vi "UHR-Fleezers Control (host) - 12.5.vi"() -> ()   [LabVIEW 2012] (continued)
                                n602 = Wait (ms)(milliseconds to wait=u32 700) -> ()  [unwired: 1 out]
                                }
                                frame #2 {
                                n603 = local read "Action (%)"() -> (w916:dbl)
                                n604 = Absolute Value(x=w916) -> (abs(x)=w915:dbl)
                                n605 = Greater?(x=w915, y=70.0) -> (0:w913:bool)
                                n606 = property on="Remove Action Offset" class="Bool (strict)"("Val(Sgnl)"=w913) -> ()  [unwired: 2 in, 2 out]
                                }
                                frame #3 {
                                n607 = for {
                                N: 4 -> [_]
                                n608 = flat-sequence {
                                frame #0 {
                                n609 = Wait (ms)(milliseconds to wait=u32 500) -> ()  [unwired: 1 out]
                                }
                                frame #1 {
                                n610 = local read "Action (%)"() -> (w922:dbl)
                                n611 = Absolute Value(x=w922) -> (abs(x)=w921:dbl)
                                n612 = Greater?(x=w921, y=70.0) -> (0:w919:bool)
                                n613 = property on="Remove Action Offset" class="Bool (strict)"("Val(Sgnl)"=w919) -> ()  [unwired: 2 in, 2 out]
                                }
                                }
                                }
                                }
                                frame #4 {
                                n614 = local read "Shift confocal"() -> (w927:bool)
                                n615 = local read "Mean"() -> (w929:dbl)
                                n616 = Greater?(x=w929, y=11.0) -> (0:w926:bool)
                                n617 = Not(x=w926) -> (.not. x?=w925:bool)
                                n618 = And(x=w926, y=w927) -> (x .and. y?=w924:bool)
                                n619 = And(x=w925, y=w927) -> (x .and. y?=w923:bool)
                                n620 = case shown="True" w924 {
                                frame False {
                                }
                                frame True {
                                n621 = local read "Confocal Y 2 (V)"() -> (w933:dbl)
                                n622 = local read "Confocal X 2 (V)"() -> (w932:dbl)
                                n623 = property on="AO2" class="Slide (strict)"("Val(Sgnl)"=w932) -> ()  [unwired: 2 in, 2 out]
                                n624 = property on="AO1" class="Slide (strict)"("Val(Sgnl)"=w933) -> ()  [unwired: 2 in, 2 out]
                                }
                                }
                                n625 = case shown="True" w923 {
                                frame False {
                                }
                                frame True {
                                n626 = local read "Confocal X 1 (V)"() -> (w930:dbl)
                                n627 = local read "Confocal Y 1 (V)"() -> (w931:dbl)
                                n628 = property on="AO1" class="Slide (strict)"("Val(Sgnl)"=w931) -> ()  [unwired: 2 in, 2 out]
                                n629 = property on="AO2" class="Slide (strict)"("Val(Sgnl)"=w930) -> ()  [unwired: 2 in, 2 out]
                                }
                                }
                                }
                                frame #5 {
                                n630 = Wait (ms)(milliseconds to wait=u32 1500) -> ()  [unwired: 1 out]
                                }
                                frame #6 {
                                n631 = property on="Rem fb disp offset" class="Bool (strict)"("Val(Sgnl)"=TRUE ("Value (Signaling)")) -> ()  [unwired: 2 in, 2 out]
                                }
                                }
                                }
                                frame True {
                                n632 = flat-sequence {
                                tunnel: w936 -> [w937]
                                frame #0 {
                                n633 = property on="Trap Delta (MHz)" class="DigNum (strict)"("Val(Sgnl)"=w937) -> ()  [unwired: 2 in, 2 out]
                                }
                                frame #1 {
                                n634 = Wait (ms)(milliseconds to wait=u32 500) -> ()  [unwired: 1 out]
                                }
                                frame #2 {
                                n635 = local read "Shift confocal"() -> (w943:bool)
                                n636 = local read "Mean"() -> (w945:dbl)
                                n637 = Greater?(x=w945, y=11.0) -> (0:w942:bool)
                                n638 = Not(x=w942) -> (.not. x?=w941:bool)
                                n639 = And(x=w942, y=w943) -> (x .and. y?=w940:bool)
                                n640 = And(x=w941, y=w943) -> (x .and. y?=w939:bool)
                                n641 = case shown="True" w940 {
                                frame False {
                                }
                                frame True {
                                n642 = local read "Confocal Y 2 (V)"() -> (w949:dbl)
                                n643 = local read "Confocal X 2 (V)"() -> (w948:dbl)
                                n644 = property on="AO2" class="Slide (strict)"("Val(Sgnl)"=w948) -> ()  [unwired: 2 in, 2 out]
                                n645 = property on="AO1" class="Slide (strict)"("Val(Sgnl)"=w949) -> ()  [unwired: 2 in, 2 out]
                                }
                                }
                                n646 = case shown="True" w939 {
                                frame False {
                                }
                                frame True {
                                n647 = local read "Confocal Y 1 (V)"() -> (w947:dbl)
                                n648 = local read "Confocal X 1 (V)"() -> (w946:dbl)
                                n649 = property on="AO2" class="Slide (strict)"("Val(Sgnl)"=w946) -> ()  [unwired: 2 in, 2 out]
                                n650 = property on="AO1" class="Slide (strict)"("Val(Sgnl)"=w947) -> ()  [unwired: 2 in, 2 out]
                                }
                                }
                                }
                                }
                                }
                                }
                                }
                                }
                                }
                                }
                                n651 = local read "Messages"() -> (w895:string)
                                n652 = Subtract(x=w887, y=w886) -> (x-y=w893:dbl)
                                "Duration (s)" <- w893
                                n653 = Number To Decimal String(number=w893, width (-)=i16 0) -> (decimal integer string=w891:string)
                                n654 = Concatenate Strings(w891, " s fluorescence event." ("string")) -> (w889:string)
                                n655 = call "Update messages.vi"("Message to add"=w889, "Old message string"=w895) -> ("New message string"=w894:string)
                                n656 = local write "Reset Force"(FALSE ("Reset Force")) -> ()
                                n657 = local write "Waiting"(TRUE ("Waiting")) -> ()
                                n658 = local write "Messages"(w894) -> ()
                                n659 = local write "Fl. High"(FALSE ("Fl. High")) -> ()
                                n660 = call <vilib>:"Beep.vi"() -> ()  [unwired: 3 in, 9 out]
                                }
                                }
                                n661 = node-c288() -> ()  [unwired: 2 out]
                              }
                              n662 = node-c288(w863) -> ()  [unwired: 1 out]
                            }
                          }
                        }
                      }
                      n663 = local read "Trap Delta (MHz)"() -> (w778:dbl)
                      n664 = local read "Trap Pos FB SP"() -> (w773:fxp<+/-,16,1>)
                    }
                  }
                }
                frame #1 {
                  n665 = local read "Stop All"() -> (w959:bool)
                  n666 = local read "Fl. Triggered..."() -> (w957:bool)
                  n667 = Not(x=w957) -> (.not. x?=w958:bool)
                  n668 = Or(x=w958, y=w959) -> (x .or. y?=w956:bool)
                }
              }
              n669 = case shown="True" w550 {
                frame False {
                }
                frame True {
                  n670 = local read "Confocal Y 1 (V)"() -> (w560:dbl)
                  n671 = local read "Confocal X 1 (V)"() -> (w559:dbl)
                  n672 = property on="AO2" class="Slide (strict)"("Val(Sgnl)"=w559) -> ()  [unwired: 2 in, 2 out]
                  n673 = property on="AO1" class="Slide (strict)"("Val(Sgnl)"=w560) -> ()  [unwired: 2 in, 2 out]
                }
              }
              n674 = case shown="True" w550 {
                frame False {
                }
                frame True {
                  w558 = FALSE ("Fl. High")
                  n675 = local write "Waiting"(w558) -> ()
                  n676 = local write "Fl. High"(w558) -> ()
                }
              }
              n677 = node-c288() -> ()  [unwired: 2 out]
            }
            n678 = node-c288(w548) -> ()  [unwired: 1 out]
          }
        }
      }
      event "Stop All": Value Change {
        n679 = event-data() -> ()  [unwired: 7 out]
        n680 = local read "Stop All"() -> (w964:bool)
      }
    }
    n681 = node-c288() -> ()  [unwired: 2 out]
  }
  n682 = timed-loop "Run Scripts, including: stage motion" {
    tunnel: w119 -> [w972]
    tunnel: w118 -> [w973]
    tunnel: [w973] -> w117
    tunnel: [w972] -> w116
    timing: w114 -> [_]
    timing-out: [_] -> w113
    tunnel: w100 -> [w971]
    tunnel: w101 -> [w970]
    tunnel: w72 -> [w967]
    tunnel: w71 -> [w966]
    tunnel: w70 -> [w968]
    tunnel: w69 -> [w969]
    tunnel: w2 -> [w965]
    stop <- w974 stop-if-true
    n683 = node-c288() -> ()  [unwired: 1 in, 1 out]
    n684 = event shown="[20] \"Stop All\": Value Change" {
      selector: _ -> [_ _ _ _ _ _ _ _ _ _ _ _ _ _ _ _ _ _ _ _ _]
      dyn-events: _ -> [_ _ _ _ _ _ _ _ _ _ _ _ _ _ _ _ _ _ _ _ _]
      timeout: _ -> [_ _ _ _ _ _ _ _ _ _ _ _ _ _ _ _ _ _ _ _ _]
      tunnel: ["Set Position" "Move to Position" _ _ _ _ "Read Harvard" _ _ _ _ _ _ "Got ADig bead" "Force FB Data\nScript" _ "Got DNA bead" "Take Stepping Data" _ "Take Detection Laser\nImage" _] -> _
      tunnel: [_ _ _ _ _ _ _ _ _ _ _ _ _ _ _ _ _ _ _ _ w1626] -> w974
      tunnel: w972 -> [w992 w1000 w1013 w1043 _ _ _ w1117 w1157 w1238 w1267 w1399 w1425 _ w1461 _ _ _ _ _ _]
      tunnel: w973 -> [w993 w1001 w1014 w1044 _ _ _ w1118 w1158 w1239 w1268 w1400 w1426 _ w1462 _ _ _ _ _ _]
      tunnel: w971 -> [_ _ _ _ _ _ w1102 _ _ _ _ _ _ _ _ _ _ _ _ _ _]
      tunnel: w970 -> [_ _ _ _ _ _ w1101 _ _ _ _ _ _ _ _ _ _ _ _ _ _]
      tunnel: w969 -> [_ _ _ _ _ _ _ _ _ _ _ _ _ _ _ _ _ _ _ _ _]
      tunnel: w968 -> [_ _ _ _ _ _ _ _ _ _ _ _ _ _ _ _ _ _ _ _ _]
      tunnel: w967 -> [_ _ _ _ _ _ _ _ _ _ _ _ _ _ _ _ _ _ _ _ _]
      tunnel: w966 -> [_ _ _ _ _ _ _ _ _ _ _ _ _ _ _ _ _ _ _ _ _]
      tunnel: w965 -> [_ _ _ _ w1071 w1092 _ _ _ _ _ _ _ _ _ _ _ _ _ _ w1625]
      event "Set Position", "Set Position 2", "Set Position 3", "Set Position 4", "Set Position 5", "Set Position 1": Value Change {
        n685 = event-data() -> ()  [unwired: 1 in, 5 out]
        n686 = Build Array("Set Position 1", "Set Position 2", "Set Position 3", "Set Position 4", "Set Position 5") -> (w991:bool[])
        n687 = Boolean Array To Number(Boolean array=w991) -> (number=w990:u32)
        n688 = Logarithm Base 2(1:w990) -> (0:w982:dbl)
        n689 = call "Read Stage Position.vi"("error in"=w992, "VISA resource name in"=w993) -> ("Current Position"=w997:cluster{dbl, dbl, dbl}, "error out"=w996:errorcluster)  [unwired: 2 out]
        n690 = Decrement(x="Position") -> (x-1=w980:dbl)
        n691 = Greater Or Equal?(x=w982, y=0.0) -> (x >= y?=w983:bool)
        n692 = Cluster To Array(cluster=w997) -> (array=w994:dbl[])
        n693 = local write "Stage Control Serial Error"(w996) -> ()
        n694 = Select(t=w982, s=w983, f=w980) -> (s? t:f=w979:dbl)
        n695 = Increment(x=w979) -> (x+1=w978:dbl)
        n696 = Build Array (concatenate)(w978, w994) -> (w977:dbl[])
        n697 = Replace Array Subset(array="Saved Stage Positions", new element=w977, index (row)=w979) -> (w995:dbl[][])  [unwired: 1 in]
        n698 = local write "Saved Stage Positions"(w995) -> ()
      }
      event "Move to Position": Value Change {
        n699 = event-data() -> ()  [unwired: 1 in, 5 out]
        n700 = flat-sequence {
          tunnel: w1001 -> [w1005]
          tunnel: w1000 -> [w1004]
          frame #0 {
            n701 = local read "Saved Stage Positions"() -> (w1007:dbl[][])
            n702 = local read "Position"() -> (w1006:dbl)
            n703 = local write "Stage Moving"(TRUE ("Stage Moving")) -> ()
            n704 = call "move to saved stage position.vi"("error in"=w1004, "Stage VISA resource name in"=w1005, "Position"=w1006, "Saved Stage Positions"=w1007) -> ("error out"=w1003:errorcluster)  [unwired: 1 out]
            n705 = local write "Stage Control Serial Error"(w1003) -> ()
          }
          frame #1 {
            n706 = call <vilib>:"Beep.vi"() -> ()  [unwired: 3 in, 9 out]
            n707 = local write "Stage Moving"(FALSE ("Stage Moving")) -> ()
          }
        }
      }
      event "Move Cap. 1 (DNA Bottom)": Value Change {
        n708 = event-data() -> ()  [unwired: 1 in, 5 out]
        n709 = local write "Move Cap. 1 (DNA Bottom)"(FALSE ("Move Cap. 1 (DNA Right)")) -> ()
        n710 = flat-sequence {
          tunnel: w1013 -> [w1016]
          tunnel: w1014 -> [w1017]
          tunnel: [w1017] -> w1011
          tunnel: [w1016] -> w1010
          tunnel: w1011 -> [w1019]
          tunnel: w1010 -> [w1018]
          frame #0 {
            n711 = property on="Sample Channel\nFlow" class="Bool (strict)"("Val(Sgnl)"="Cap 1 Samp Flow ON") -> ()  [unwired: 2 in, 2 out]
          }
          frame #1 {
            n712 = local read "Saved Stage Positions"() -> (w1029:dbl[][])
            n713 = local write "Stage Moving"(TRUE ("Stage Moving")) -> ()
            n714 = Array Subset(array=w1029, index (row)=0 ("index"), length (row)=1 ("length"), index (col)=1 ("index"), length (col)=3 ("length")) -> (w1026:dbl[][])
            n715 = Reshape Array(w1026, 3 ("dimension size")) -> (w1024:dbl[])
            n716 = Array To Cluster(array=w1024) -> (cluster=w1023:cluster{"[0]":dbl, "[1]":dbl, "[2]":dbl})
            n717 = call "Set Stage Position.vi"("Position"=w1023, "error in"=w1018, "VISA resource name in"=w1019) -> ("error out"=w1022:errorcluster)  [unwired: 2 out]
            n718 = local write "Stage Control Serial Error"(w1022) -> ()
          }
          frame #2 {
            n719 = local write "Stage Moving"(FALSE ("Stage Moving")) -> ()
            n720 = case shown="True" "Cap 1 Flow ON" {
              frame False {
              }
              frame True {
                n721 = property on="Inject Pump 1" class="Bool (strict)"("Val(Sgnl)"=TRUE ("Value (Signaling)")) -> ()  [unwired: 2 in, 2 out]
              }
            }
            n722 = call <vilib>:"Beep.vi"() -> ()  [unwired: 3 in, 9 out]
          }
          frame #3 {
            n723 = property on="Sample Channel\nFlow" class="Bool (strict)"("Val(Sgnl)"=FALSE ("Value (Signaling)")) -> ()  [unwired: 2 in, 2 out]
            n724 = local read "Cap. 2 BD T1?\n(ADig T1, DNA T2)"() -> (w1036:bool)
            n725 = case shown="True" w1036 {
              tunnel: "Cap 1 T ON" -> [w1038 w1039]
              frame False {
                n726 = property on="Trap 1 (ON/OFF)" class="Bool (strict)"("Val(Sgnl)"=w1038) -> ()  [unwired: 2 in, 2 out]
              }
              frame True {
                n727 = property on="Trap 2 (ON/OFF)" class="Bool (strict)"("Val(Sgnl)"=w1039) -> ()  [unwired: 2 in, 2 out]
              }
            }
            n728 = property on="Got DNA bead" class="Bool"("Key Focus"=TRUE) -> ()  [unwired: 2 in, 2 out]
          }
        }
      }
      event "Move Cap. 2 (ADig Top)": Value Change {
        n729 = event-data() -> ()  [unwired: 1 in, 5 out]
        n730 = local write "Move Cap. 2 (ADig Top)"(FALSE ("Move Cap. 2 (ADig Left)")) -> ()
        n731 = flat-sequence {
          tunnel: w1043 -> [w1046]
          tunnel: w1044 -> [w1047]
          tunnel: [w1047] -> w1041
          tunnel: [w1046] -> w1040
          tunnel: w1041 -> [w1050]
          tunnel: w1040 -> [w1049]
          frame #0 {
            n732 = property on="Sample Channel\nFlow" class="Bool (strict)"("Val(Sgnl)"="Cap 2 Samp Flow ON") -> ()  [unwired: 2 in, 2 out]
          }
          frame #1 {
            w1048 = FALSE ("Value (Signaling)")
            n733 = local read "Saved Stage Positions"() -> (w1060:dbl[][])
            n734 = local write "Stage Moving"(TRUE ("Stage Moving")) -> ()
            n735 = Array Subset(array=w1060, index (row)=1 ("index"), length (row)=1 ("length"), index (col)=1 ("index"), length (col)=3 ("length")) -> (w1057:dbl[][])
            n736 = Reshape Array(w1057, 3 ("dimension size")) -> (w1055:dbl[])
            n737 = property on="Trap 1 (ON/OFF)" class="Bool (strict)"("Val(Sgnl)"=w1048) -> ()  [unwired: 2 in, 2 out]
            n738 = property on="Trap 1 (ON/OFF)" class="Bool (strict)"("Val(Sgnl)"=w1048) -> ()  [unwired: 2 in, 2 out]
            n739 = Array To Cluster(array=w1055) -> (cluster=w1054:cluster{"[0]":dbl, "[1]":dbl, "[2]":dbl})
            n740 = call "Set Stage Position.vi"("Position"=w1054, "error in"=w1049, "VISA resource name in"=w1050) -> ("error out"=w1053:errorcluster)  [unwired: 2 out]
            n741 = local write "Stage Control Serial Error"(w1053) -> ()
          }
          frame #2 {
            n742 = local write "Stage Moving"(FALSE ("Stage Moving")) -> ()
            n743 = call <vilib>:"Beep.vi"() -> ()  [unwired: 3 in, 9 out]
            n744 = case shown="True" "Cap 2 Flow ON" {
              frame False {
              }
              frame True {
                n745 = property on="Inject Pump 3" class="Bool (strict)"("Val(Sgnl)"=TRUE ("Value (Signaling)")) -> ()  [unwired: 2 in, 2 out]
              }
            }
          }
          frame #3 {
            n746 = property on="Sample Channel\nFlow" class="Bool (strict)"("Val(Sgnl)"=FALSE ("Value (Signaling)")) -> ()  [unwired: 2 in, 2 out]
            n747 = case shown="False" "Cap. 2 BD T1?\n(ADig T1, DNA T2)" {
              tunnel: "Cap 2 T ON" -> [w1069 w1070]
              frame False {
                n748 = property on="Trap 2 (ON/OFF)" class="Bool (strict)"("Val(Sgnl)"=w1069) -> ()  [unwired: 2 in, 2 out]
              }
              frame True {
                n749 = property on="Trap 1 (ON/OFF)" class="Bool (strict)"("Val(Sgnl)"=w1070) -> ()  [unwired: 2 in, 2 out]
              }
            }
            n750 = property on="Got ADig bead" class="Bool"("Key Focus"=TRUE) -> ()  [unwired: 2 in, 2 out]
          }
        }
      }
      event "Initialize Blue Laser": Value Change {
        n751 = event-data() -> ()  [unwired: 1 in, 5 out]
        n752 = flat-sequence {
          tunnel: w1071 -> [w1090]
          frame #0 {
            n753 = Concatenate Strings("slmp ", "Modulation\nPower (mW)") -> (w1089:string)
            n754 = call "serial write macro.vi"("String"=w1089, "Delay (ms)"="Delay (ms)", "VISA resource name"=w1090) -> ("read buffer"=w1078:string, "error out"=w1079:errorcluster, "VISA resource name out"=w1086:refnum<visa-resource-name>)
            n755 = local write "read blue buffer"(w1078) -> ()
            n756 = local write "Blue Error Out"(w1079) -> ()
            n757 = call "serial write macro.vi"("String"="sdmes 1", "Delay (ms)"="Delay (ms)", "VISA resource name"=w1086) -> ("read buffer"=w1076:string, "error out"=w1077:errorcluster, "VISA resource name out"=w1084:refnum<visa-resource-name>)
            n758 = local write "Blue Error Out"(w1077) -> ()
            n759 = local write "read blue buffer"(w1076) -> ()
            n760 = call "serial write macro.vi"("String"="sames 1", "Delay (ms)"="Delay (ms)", "VISA resource name"=w1084) -> ("read buffer"=w1073:string, "error out"=w1075:errorcluster, "VISA resource name out"=w1081:refnum<visa-resource-name>)
            n761 = local write "read blue buffer"(w1073) -> ()
            n762 = local write "Blue Error Out"(w1075) -> ()
            n763 = call "serial write macro.vi"("String"="l1", "Delay (ms)"="Delay (ms)", "VISA resource name"=w1081) -> ("read buffer"=w1072:string, "error out"=w1074:errorcluster)  [unwired: 1 out]
            n764 = local write "read blue buffer"(w1072) -> ()
            n765 = local write "Blue Error Out"(w1074) -> ()
          }
          frame #1 {
            n766 = local write "Initialize Blue Laser"(FALSE ("Initialize")) -> ()
          }
        }
      }
      event "Send string\nto Blue Laser": Value Change {
        n767 = event-data() -> ()  [unwired: 1 in, 5 out]
        n768 = flat-sequence {
          tunnel: w1092 -> [w1097]
          frame #0 {
            n769 = local read "Delay (ms)"() -> (w1094:i32)
            n770 = call "serial write macro.vi"("String"="command string", "Delay (ms)"=w1094, "VISA resource name"=w1097) -> ("read buffer"=w1095:string, "error out"=→"Blue Error Out":errorcluster)  [unwired: 1 out]
            "read blue buffer" <- w1095
            n771 = String Length(string=w1095) -> (length=→"length":i32)
            "command string sent" <- "command string"
          }
          frame #1 {
            n772 = local write "Send string\nto Blue Laser"(FALSE ("Send string")) -> ()
          }
        }
      }
      event "Read Harvard": Value Change {
        n773 = event-data() -> ()  [unwired: 1 in, 5 out]
        n774 = Concatenate Strings("write buffer", "\r") -> (w1104:string)
        n775 = VISA Write(VISA resource name=w1102, write buffer=w1104, error in (no error)=w1101) -> (VISA resource name out=w1113:refnum<visa-resource-name>, error out=w1112:errorcluster)  [unwired: 1 out]
        n776 = stacked-sequence {
          tunnel: [w1116] -> w1111
          tunnel: w1113 -> [w1116]
          tunnel: w1112 -> [w1115]
          tunnel: [w1115] -> w1106
          frame #0 {
            n777 = Wait (ms)(milliseconds to wait=50) -> ()  [unwired: 1 out]
          }
        }
        n778 = property class="Instr"(reference=w1111, error in=w1106) -> (reference out=w1110:refnum<visa-resource-name>, error out=w1108:errorcluster, "Serial Settings:Number of Bytes at Serial Port"=w1109:u32)
        "Serial Settings:Number of Bytes at Serial Port" <- w1109
        n779 = VISA Read(VISA resource name=w1110, byte count=w1109, error in (no error)=w1108) -> (read buffer=w1107:string)  [unwired: 3 out]
        "read buffer" <- w1107
        n780 = Fract/Exp String To Number(string=w1107) -> ()  [unwired: 5 out]
      }
      event "+z", "-z": Value Change {
        n781 = event-data() -> ()  [unwired: 1 in, 5 out]
        n782 = flat-sequence {
          tunnel: w1117 -> [w1139]
          tunnel: w1118 -> [w1119]
          frame #0 {
            n783 = call "Read Stage Position.vi"("error in"=w1139, "VISA resource name in"=w1119) -> ("Current Position"=w1124:cluster{dbl, dbl, dbl}, "error out"=w1137:errorcluster, "VISA resource name out"=w1138:refnum<visa-resource-name>)  [unwired: 1 out]
            n784 = local read "Saved Stage Positions"() -> (w1148:dbl[][])
            n785 = Divide(x="z nudge increment (um)", y=1000.0) -> (x/y=w1136:dbl)
            n786 = Boolean To (0,1)(Boolean="+z") -> (0, 1=w1128:i16)
            n787 = Boolean To (0,1)(Boolean="-z") -> (0, 1=w1129:i16)
            n788 = Array Subset(array=w1148, index (row)=1 ("index"), length (row)=1 ("length"), index (col)=1 ("index"), length (col)=3 ("length")) -> (w1145:dbl[][])
            n789 = Multiply(x=w1128, y=w1136) -> (x*y=w1132:dbl)
            n790 = Multiply(x=w1129, y=w1136) -> (x*y=w1130:dbl)
            n791 = Unbundle(w1124) -> (w1122:dbl, w1121:dbl, w1125:dbl)
            n792 = Negate(x=w1130) -> (-x=w1131:dbl)
            n793 = Reshape Array(w1145, 3 ("dimension size")) -> (w1143:dbl[])
            n794 = Add(x=w1132, y=w1131) -> (x+y=w1133:dbl)
            n795 = Array To Cluster(array=w1143) -> ()  [unwired: 1 out]
            n796 = Add(x=w1133, y=w1125) -> (x+y=w1123:dbl)
            n797 = Bundle(cluster=w1124, w1122, w1121, w1123) -> (w1120:cluster{dbl, dbl, dbl})
            n798 = call "Set Stage Position.vi"("Position"=w1120, "error in"=w1137, "VISA resource name in"=w1138) -> ("error out"=w1142:errorcluster)  [unwired: 2 out]
            n799 = local write "Stage Moving"(TRUE ("Stage Moving")) -> ()
            n800 = local write "Stage Control Serial Error"(w1142) -> ()
          }
          frame #1 {
            n801 = local write "Stage Moving"(FALSE ("Stage Moving")) -> ()
            n802 = call <vilib>:"Beep.vi"() -> ()  [unwired: 3 in, 9 out]
          }
        }
      }
      event "Cal/Data Acq. Spot": Value Change {
        n803 = event-data() -> ()  [unwired: 1 in, 5 out]
        n804 = flat-sequence {
          tunnel: w1157 -> [w1161]
          tunnel: w1158 -> [w1162]
          tunnel: [w1162] -> w1154
          tunnel: [w1161] -> w1153
          tunnel: w1154 -> [w1167]
          tunnel: w1153 -> [w1166]
          tunnel: ["Cal @ (MHz)"] -> w1151
          tunnel: [w1171] -> w1155
          tunnel: w1151 -> [w1171]
          tunnel: w1155 -> [w1180]
          tunnel: ["W/ Offset 1"] -> w1152
          tunnel: w1155 -> [w1201]
          tunnel: w1152 -> [w1199]
          frame #0 {
            n805 = property on="Sample Channel\nFlow" class="Bool (strict)"("Val(Sgnl)"="Daq spot flow on") -> ()  [unwired: 2 in, 2 out]
            n806 = Wait (ms)(milliseconds to wait=u32 250) -> ()  [unwired: 1 out]
          }
          frame #1 {
            n807 = local read "Saved Stage Positions"() -> (w1164:dbl[][])
            n808 = property on="Trap Delta (MHz)" class="DigNum (strict)"("Val(Sgnl)"="Cal @ (MHz)") -> ()  [unwired: 2 in, 2 out]
            n809 = local write "Stage Moving"(TRUE ("Stage Moving")) -> ()
            n810 = call "move to saved stage position.vi"("error in"=w1166, "Stage VISA resource name in"=w1167, "Position"="Cal Stage Position", "Saved Stage Positions"=w1164) -> ("error out"=w1165:errorcluster)  [unwired: 1 out]
            n811 = local write "Stage Control Serial Error"(w1165) -> ()
          }
          frame #2 {
            n812 = local write "Stage Moving"(FALSE ("Stage Moving")) -> ()
            n813 = property on="Sample Channel\nFlow" class="Bool (strict)"("Val(Sgnl)"="Flow ON during cal?") -> ()  [unwired: 2 in, 2 out]
            n814 = call <vilib>:"Beep.vi"() -> ()  [unwired: 3 in, 9 out]
          }
          frame #3 {
            n815 = Wait (ms)(milliseconds to wait=u32 1000) -> ()  [unwired: 1 out]
          }
          frame #4 {
            n816 = property on="Save Calibration" class="Bool (strict)"("Val(Sgnl)"=TRUE ("Value (Signaling)")) -> ()  [unwired: 2 in, 2 out]
          }
          frame #5 {
            n817 = Wait (ms)(milliseconds to wait=u32 2000) -> ()  [unwired: 1 out]
          }
          frame #6 {
            # "Check to see if \nsaving done"
            n818 = while {
              stop <- w1176 stop-if-true
              n819 = local read "Saving..."() -> (w1177:bool)
              n820 = Wait (ms)(milliseconds to wait=u32 100) -> ()  [unwired: 1 out]
              n821 = Not(x=w1177) -> (.not. x?=w1176:bool)
            }
          }
          frame #7 {
            n822 = case shown="True" "W/ Offset 1" {
              tunnel: w1180 -> [_ w1181]
              frame False {
              }
              frame True {
                n823 = stacked-sequence {
                  tunnel: w1181 -> [_ _ _ _ _ _ _ w1198]
                  frame #0 {
                    n824 = property on="Trap Delta (MHz)" class="DigNum (strict)"("Val(Sgnl)"="Offset 1 Start (MHz)") -> ()  [unwired: 2 in, 2 out]
                    n825 = Replace Array Subset(array=u32[] [0] ("Index Values"), new element="Offset 1 Set", index=0) -> (w1182:u32[])
                    n826 = property on="Saved AOD Raster Scan Parameter Sets" class="Arr (strict)"("Index Values"=w1182) -> ()  [unwired: 2 in, 2 out]
                  }
                  frame #1 {
                    n827 = Wait (ms)(milliseconds to wait=u32 200) -> ()  [unwired: 1 out]
                  }
                  frame #2 {
                    n828 = property on="Load parameters" class="Bool (strict)"("Val(Sgnl)"=TRUE ("Value (Signaling)")) -> ()  [unwired: 2 in, 2 out]
                  }
                  frame #3 {
                    n829 = Wait (ms)(milliseconds to wait=u32 200) -> ()  [unwired: 1 out]
                  }
                  frame #4 {
                    n830 = property on="Trap Raster Scan" class="Bool (strict)"("Val(Sgnl)"=TRUE ("Value (Signaling)")) -> ()  [unwired: 2 in, 2 out]
                  }
                  frame #5 {
                    n831 = Wait (ms)(milliseconds to wait=u32 2000) -> ()  [unwired: 1 out]
                  }
                  frame #6 {
                    n832 = while {
                      stop <- w1195 stop-if-true
                      n833 = local read "Raster Scanning..."() -> (w1197:bool)
                      n834 = local read "Saving..."() -> (w1193:bool)
                      n835 = Wait (ms)(milliseconds to wait=u32 100) -> ()  [unwired: 1 out]
                      n836 = Not(x=w1193) -> (.not. x?=w1192:bool)
                      n837 = Not(x=w1197) -> (.not. x?=w1194:bool)
                      n838 = And(x=w1194, y=w1192) -> (x .and. y?=w1195:bool)
                    }
                  }
                  frame #7 {
                    n839 = property on="Trap Delta (MHz)" class="DigNum (strict)"("Val(Sgnl)"=w1198) -> ()  [unwired: 2 in, 2 out]
                  }
                }
              }
            }
          }
          frame #8 {
            n840 = local read "Save ave N"() -> (w1200:dbl)
            n841 = case shown="False" "W/ Offset 2" {
              tunnel: w1201 -> [_ w1208]
              tunnel: w1200 -> [_ w1207]
              tunnel: w1199 -> [w1203 _]
              frame False {
                n842 = case shown="False" w1203 {
                  frame False {
                    n843 = Multiply(x="Cal read wait (s)", y=u32 1000 ("milliseconds to wait")) -> (x*y=w1205:u32)
                    n844 = Wait (ms)(milliseconds to wait=w1205) -> ()  [unwired: 1 out]
                  }
                  frame True {
                  }
                }
              }
              frame True {
                n845 = stacked-sequence {
                  tunnel: w1208 -> [_ _ _ _ _ _ _ _ _ w1229 _ _]
                  tunnel: w1207 -> [_ _ _ _ _ _ _ _ _ w1227 _ _]
                  frame #0 {
                    n846 = property on="Save ave N" class="DigNum (strict)"("Val(Sgnl)"=1.0 ("Value (Signaling)")) -> ()  [unwired: 2 in, 2 out]
                  }
                  frame #1 {
                    n847 = Wait (ms)(milliseconds to wait=u32 500) -> ()  [unwired: 1 out]
                  }
                  frame #2 {
                    n848 = property on="Trap Delta (MHz)" class="DigNum (strict)"("Val(Sgnl)"="Offset 2 Start (MHz)") -> ()  [unwired: 2 in, 2 out]
                    n849 = Replace Array Subset(array=u32[] [0] ("Index Values"), new element="Offset 2 Set", index=0) -> (w1213:u32[])
                    n850 = property on="Saved AOD Raster Scan Parameter Sets" class="Arr (strict)"("Index Values"=w1213) -> ()  [unwired: 2 in, 2 out]
                  }
                  frame #3 {
                    n851 = Wait (ms)(milliseconds to wait=u32 500) -> ()  [unwired: 1 out]
                  }
                  frame #4 {
                    n852 = property on="Load parameters" class="Bool (strict)"("Val(Sgnl)"=TRUE ("Value (Signaling)")) -> ()  [unwired: 2 in, 2 out]
                  }
                  frame #5 {
                    n853 = Wait (ms)(milliseconds to wait=u32 500) -> ()  [unwired: 1 out]
                  }
                  frame #6 {
                    n854 = property on="Trap Raster Scan" class="Bool (strict)"("Val(Sgnl)"=TRUE ("Value (Signaling)")) -> ()  [unwired: 2 in, 2 out]
                  }
                  frame #7 {
                    n855 = Wait (ms)(milliseconds to wait=u32 2000) -> ()  [unwired: 1 out]
                  }
                  frame #8 {
                    n856 = while {
                      stop <- w1222 stop-if-true
                      n857 = local read "Raster Scanning..."() -> (w1225:bool)
                      n858 = local read "Saving..."() -> (w1223:bool)
                      n859 = Wait (ms)(milliseconds to wait=u32 100) -> ()  [unwired: 1 out]
                      n860 = Not(x=w1223) -> (.not. x?=w1221:bool)
                      n861 = Not(x=w1225) -> (.not. x?=w1224:bool)
                      n862 = And(x=w1224, y=w1221) -> (x .and. y?=w1222:bool)
                    }
                  }
                  frame #9 {
                    n863 = property on="Trap Delta (MHz)" class="DigNum (strict)"("Val(Sgnl)"=w1229) -> ()  [unwired: 2 in, 2 out]
                    n864 = property on="Saved AOD Raster Scan Parameter Sets" class="Arr (strict)"("Index Values"=u32[] [0]) -> ()  [unwired: 2 in, 2 out]
                    n865 = property on="Save ave N" class="DigNum (strict)"("Val(Sgnl)"=w1227) -> ()  [unwired: 2 in, 2 out]
                  }
                  frame #10 {
                    n866 = Wait (ms)(milliseconds to wait=u32 500) -> ()  [unwired: 1 out]
                  }
                  frame #11 {
                    n867 = property on="Load parameters" class="Bool (strict)"("Val(Sgnl)"=TRUE ("Value (Signaling)")) -> ()  [unwired: 2 in, 2 out]
                  }
                }
              }
            }
          }
          frame #9 {
            n868 = property on="Read Cal" class="Bool (strict)"("Val(Sgnl)"=TRUE ("Value (Signaling)")) -> ()  [unwired: 2 in, 2 out]
          }
          frame #10 {
            n869 = Wait (ms)(milliseconds to wait=u32 1000) -> ()  [unwired: 1 out]
          }
          frame #11 {
            n870 = property on="Fish for Tether" class="Bool (strict)"("Val(Sgnl)"=TRUE ("Value (Signaling)")) -> ()  [unwired: 2 in, 2 out]
          }
        }
        n871 = local write "Cal/Data Acq. Spot"(FALSE ("Cal/Data Acq. Spot")) -> ()
      }
      event "Dump Beads": Value Change {
        n872 = event-data() -> ()  [unwired: 1 in, 5 out]
        n873 = flat-sequence {
          tunnel: ["Dump spot flow on?"] -> w1235
          tunnel: [w1246] -> w1236
          tunnel: w1235 -> [w1246]
          tunnel: w1239 -> [w1251]
          tunnel: w1238 -> [w1250]
          tunnel: [w1248] -> w1237
          tunnel: w1236 -> [w1248]
          tunnel: w1237 -> [w1261]
          frame #0 {
            w1240 = FALSE ("Value (Signaling)")
            n874 = local read "Saving..."() -> (w1242:bool)
            n875 = local write "Dump Beads"(FALSE ("Dump Beads")) -> ()
            n876 = property on="Inject Pump 3" class="Bool (strict)"("Val(Sgnl)"=w1240) -> ()  [unwired: 2 in, 2 out]
            n877 = property on="Inject Pump 1" class="Bool (strict)"("Val(Sgnl)"=w1240) -> ()  [unwired: 2 in, 2 out]
            n878 = local write "Stop Saving"(w1242) -> ()
          }
          frame #1 {
            w1243 = FALSE ("Fl. Triggered...")
            n879 = case shown="True" "Dump spot flow on?" {
              frame False {
              }
              frame True {
                n880 = property on="Sample Channel\nFlow" class="Bool (strict)"("Val(Sgnl)"=TRUE ("Stage Moving")) -> ()  [unwired: 2 in, 2 out]
              }
            }
            n881 = local write "Fl. Triggered..."(w1243) -> ()
            n882 = local write "Tether"(w1243) -> ()
            n883 = property on="Green Laser ON" class="Bool (strict)"("Val(Sgnl)"=w1243) -> ()  [unwired: 2 in, 2 out]
            n884 = property on="Trap Pos. FB ON" class="Bool (strict)"("Val(Sgnl)"=w1243) -> ()  [unwired: 2 in, 2 out]
            n885 = property on="Trap Trig. Fl." class="Bool (strict)"("Val(Sgnl)"=w1243) -> ()  [unwired: 2 in, 2 out]
            n886 = property on="Fl. Triggered..." class="Bool (strict)"("Val(Sgnl)"=w1243) -> ()  [unwired: 2 in, 2 out]
            n887 = property on="Dip for Protein" class="Bool (strict)"("Val(Sgnl)"=w1243) -> ()  [unwired: 2 in, 2 out]
            n888 = property on="Pause dwell" class="Bool (strict)"("Val(Sgnl)"=w1243) -> ()  [unwired: 2 in, 2 out]
          }
          frame #2 {
            n889 = property on="Trap Pos. FB Offset Factor" class="DigNum (strict)"("Val(Sgnl)"=i64 0 ("Value (Signaling)")) -> ()  [unwired: 2 in, 2 out]
          }
          frame #3 {
            n890 = local read "Saved Stage Positions"() -> (w1252:dbl[][])
            n891 = local write "Stage Moving"(TRUE ("Stage Moving")) -> ()
            n892 = Array Subset(array=w1252, index (row)=3 ("index"), length (row)=1 ("length"), index (col)=1 ("index"), length (col)=3 ("length")) -> (w1257:dbl[][])
            n893 = Reshape Array(w1257, 3 ("dimension size")) -> (w1255:dbl[])
            n894 = Array To Cluster(array=w1255) -> (cluster=w1254:cluster{"[0]":dbl, "[1]":dbl, "[2]":dbl})
            n895 = call "Set Stage Position.vi"("Position"=w1254, "error in"=w1250, "VISA resource name in"=w1251) -> ()  [unwired: 3 out]
          }
          frame #4 {
            w1262 = FALSE ("Value (Signaling)")
            n896 = case shown="True" w1261 {
              frame False {
              }
              frame True {
                n897 = property on="Sample Channel\nFlow" class="Bool (strict)"("Val(Sgnl)"=FALSE ("Stage Moving")) -> ()  [unwired: 2 in, 2 out]
              }
            }
            n898 = property on="Trap 1 (ON/OFF)" class="Bool (strict)"("Val(Sgnl)"=w1262) -> ()  [unwired: 2 in, 2 out]
            n899 = property on="Trap 2 (ON/OFF)" class="Bool (strict)"("Val(Sgnl)"=w1262) -> ()  [unwired: 2 in, 2 out]
            n900 = call <vilib>:"Beep.vi"() -> ()  [unwired: 3 in, 9 out]
          }
          frame #5 {
            n901 = property on="Move Cap. 2 (ADig Top)" class="Bool (strict)"("Val(Sgnl)"=TRUE ("Value (Signaling)")) -> ()  [unwired: 2 in, 2 out]
            n902 = property on="Tab Control" class="TabCtl (strict)"("Val(Sgnl)"=T26."Status" ("Value (Signaling)")) -> ()  [unwired: 2 in, 2 out]
          }
        }
      }
      event "Dip for Protein": Value Change {
        n903 = event-data() -> ()  [unwired: 1 in, 5 out]
        n904 = case shown="True" "Dip for Protein" {
          tunnel: w1268 -> [_ w1270]
          tunnel: w1267 -> [_ w1269]
          frame False {
          }
          frame True {
            n905 = while {
              tunnel: w1270 -> [w1281]
              tunnel: w1269 -> [w1280]
              i -> [w1275]
              stop <- w1277 stop-if-true
              n906 = Increment(x=w1275) -> (x+1=→"Dip #":i32)
              n907 = flat-sequence {
                tunnel: w1280 -> [w1292]
                tunnel: w1281 -> [w1293]
                tunnel: [w1293] -> w1285
                tunnel: [w1292] -> w1284
                tunnel: [w1286] -> w1271
                tunnel: [w1298] -> w1279
                tunnel: [w1299] -> w1278
                tunnel: w1285 -> [w1300]
                tunnel: w1284 -> [w1301]
                tunnel: [w1296] -> w1272
                tunnel: w1271 -> [w1296]
                tunnel: [w1309] -> w1283
                tunnel: w1279 -> [w1309]
                tunnel: [w1308] -> w1282
                tunnel: w1278 -> [w1308]
                tunnel: [w1305] -> w1276
                tunnel: [w1304] -> w1273
                tunnel: w1272 -> [w1304]
                tunnel: w1282 -> [w1329]
                tunnel: w1283 -> [w1330]
                tunnel: w1276 -> [w1331]
                tunnel: w1273 -> [w1328]
                tunnel: [w1387] -> w1277
                frame #0 {
                  n908 = local read "Trap Pos. FB ON"() -> (w1286:bool)
                  n909 = Compound Arithmetic op=AND("Flow ON\nduring dip?", "FB OFF when \nflow ON", w1286) -> (w1287:bool)
                  n910 = case shown="True" "Move trap \nbefore dip move?" {
                    frame False {
                    }
                    frame True {
                      n911 = property on="Trap Delta (MHz)" class="DigNum (strict)"("Val(Sgnl)"="Dipping Delta (MHz)") -> ()  [unwired: 2 in, 2 out]
                    }
                  }
                  n912 = property on="Green Laser ON" class="Bool (strict)"("Val(Sgnl)"="Green ON\nbefore dip?") -> ()  [unwired: 2 in, 2 out]
                  n913 = property on="Sample Channel\nFlow" class="Bool (strict)"("Val(Sgnl)"="Flow ON\nduring dip?") -> ()  [unwired: 2 in, 2 out]
                  n914 = case shown="True" w1287 {
                    frame False {
                    }
                    frame True {
                      n915 = property on="Trap Pos. FB ON" class="Bool (strict)"("Val(Sgnl)"=FALSE ("Value (Signaling)")) -> ()  [unwired: 2 in, 2 out]
                    }
                  }
                }
                frame #1 {
                  n916 = local read "Saved Stage Positions"() -> (w1303:dbl[][])
                  n917 = local write "Cancel dwell"(FALSE ("Cancel dwell")) -> ()
                  n918 = call "move to saved stage position.vi"("error in"=w1301, "Stage VISA resource name in"=w1300, "Position"="Dip Stage \nPosition", "Saved Stage Positions"=w1303) -> ("VISA resource name out"=w1298:refnum<visa-resource-name>, "error out"=w1299:errorcluster)
                }
                frame #2 {
                  n919 = node-c288() -> (w1307:T23)  [unwired: 4 in]
                  n920 = timed-loop {
                    timing: w1307 -> [_]
                    timing-out: [_] -> w1306
                    tunnel: [w1313] -> w1305
                    i -> [w1310]
                    stop <- w1314 stop-if-true
                    n921 = node-c288() -> ()  [unwired: 1 in, 1 out]
                    n922 = Greater Or Equal?(x=w1310, y="Dip Duration (s)") -> (x >= y?=w1322:bool)
                    n923 = local read "Dip for Protein"() -> (w1315:bool)
                    n924 = local read "Dump Beads"() -> (w1312:bool)
                    n925 = local read "Cancel dwell"() -> (w1321:bool)
                    n926 = local read "Pause dwell"() -> (w1318:bool)
                    n927 = Not(x=w1315) -> (.not. x?=w1320:bool)
                    n928 = Compound Arithmetic op=OR(w1321, w1322, w1320) -> (w1319:bool)
                    n929 = Select(t=FALSE, s=w1318, f=w1319) -> (s? t:f=w1316:bool)
                    n930 = Not(x=w1312) -> (.not. x?=w1311:bool)
                    n931 = node-c288() -> ()  [unwired: 1 in, 1 out]
                    n932 = And(x=w1315, y=w1311) -> (x .and. y?=w1313:bool)
                    n933 = Or(x=w1316, y=w1312) -> (x .or. y?=w1314:bool)
                    "Dip Time (s)" <- w1310
                  }
                  n934 = node-c288(w1306) -> ()  [unwired: 1 out]
                }
                frame #3 {
                  n935 = case shown="True" w1331 {
                    tunnel: w1330 -> [_ w1336]
                    tunnel: w1329 -> [_ w1335]
                    tunnel: w1328 -> [_ w1332]
                    frame False {
                    }
                    frame True {
                      n936 = flat-sequence {
                        tunnel: w1335 -> [w1340]
                        tunnel: w1336 -> [w1341]
                        tunnel: [w1341] -> w1334
                        tunnel: [w1340] -> w1333
                        tunnel: w1332 -> [w1337]
                        tunnel: w1334 -> [w1351]
                        tunnel: w1333 -> [w1350]
                        tunnel: w1332 -> [w1359]
                        frame #0 {
                          n937 = local read "Sample Channel\nFlow"() -> (w1339:bool)
                          n938 = case shown="True" w1339 {
                            tunnel: "Flow ON \nduring return\nfrom dip?" -> [w1342 w1345]
                            tunnel: w1337 -> [_ w1344]
                            frame False {
                              n939 = case shown="True" w1342 {
                                frame False {
                                }
                                frame True {
                                n940 = property on="Sample Channel\nFlow" class="Bool (strict)"("Val(Sgnl)"=TRUE ("Value (Signaling)")) -> ()  [unwired: 2 in, 2 out]
                                }
                              }
                            }
                            frame True {
                              n941 = case shown="False" w1345 {
                                tunnel: w1344 -> [w1346 _]
                                frame False {
                                n942 = property on="Trap Pos. FB ON" class="Bool (strict)"("Val(Sgnl)"=w1346) -> ()  [unwired: 2 in, 2 out]
                                n943 = property on="Sample Channel\nFlow" class="Bool (strict)"("Val(Sgnl)"=FALSE ("Value (Signaling)")) -> ()  [unwired: 2 in, 2 out]
                                }
                                frame True {
                                }
                              }
                            }
                          }
                        }
                        frame #1 {
                          # "For turning on green laser before stage reaches lower spot"
                          n944 = case shown="True" "Green ON\nafter start\nreturn?" {
                            frame False {
                            }
                            frame True {
                              n945 = flat-sequence {
                                frame #0 {
                                n946 = Multiply(x="Green delay after \nstart return (s)", y=1000.0) -> (x*y=w1356:dbl)
                                n947 = Wait (ms)(milliseconds to wait=w1356) -> ()  [unwired: 1 out]
                                }
                                frame #1 {
                                n948 = property on="Green Laser ON" class="Bool (strict)"("Val(Sgnl)"=TRUE ("Value (Signaling)")) -> ()  [unwired: 2 in, 2 out]
                                }
                              }
                            }
                          }
                          n949 = local read "Saved Stage Positions"() -> (w1354:dbl[][])
                          n950 = local write "Cancel dwell"(FALSE ("Cancel dwell")) -> ()
                          n951 = call "move to saved stage position.vi"("error in"=w1350, "Stage VISA resource name in"=w1351, "Position"="Return Stage \nPosition", "Saved Stage Positions"=w1354) -> ("error out"=w1352:errorcluster)  [unwired: 1 out]
                          n952 = local write "Stage Control Serial Error"(w1352) -> ()
                        }
                        frame #2 {
                          n953 = property on="Trap Pos. FB ON" class="Bool (strict)"("Val(Sgnl)"=w1359) -> ()  [unwired: 2 in, 2 out]
                          n954 = case shown="True" "Green ON \nafter return?" {
                            frame False {
                            }
                            frame True {
                              n955 = property on="Green Laser ON" class="Bool (strict)"("Val(Sgnl)"=TRUE ("Value (Signaling)")) -> ()  [unwired: 2 in, 2 out]
                            }
                          }
                          n956 = case shown="True" "Move trap after return?" {
                            frame False {
                            }
                            frame True {
                              n957 = property on="Trap Delta (MHz)" class="DigNum (strict)"("Val(Sgnl)"="Dip Trap Delta 2 (MHz)") -> ()  [unwired: 2 in, 2 out]
                            }
                          }
                          n958 = case shown="True" "Save data after return?" {
                            frame False {
                            }
                            frame True {
                              n959 = property on="Start Saving" class="Bool (strict)"("Val(Sgnl)"=TRUE ("Value (Signaling)")) -> ()  [unwired: 2 in, 2 out]
                            }
                          }
                          n960 = property on="Sample Channel\nFlow" class="Bool (strict)"("Val(Sgnl)"="Flow ON\nduring daq?") -> ()  [unwired: 2 in, 2 out]
                        }
                        frame #3 {
                          n961 = node-c288() -> (w1368:T23)  [unwired: 4 in]
                          n962 = timed-loop {
                            timing: w1368 -> [_]
                            timing-out: [_] -> w1367
                            i -> [w1369]
                            stop <- w1371 stop-if-true
                            n963 = node-c288() -> ()  [unwired: 1 in, 1 out]
                            n964 = local read "Dump Beads"() -> (w1370:bool)
                            n965 = Greater Or Equal?(x=w1369, y="Dwell Duration (s)") -> (x >= y?=w1376:bool)
                            n966 = local read "Dip for Protein"() -> (w1373:bool)
                            n967 = Not(x=w1373) -> (.not. x?=w1372:bool)
                            n968 = Compound Arithmetic op=OR(w1376, "Cancel dwell", w1372) -> (w1375:bool)
                            n969 = node-c288() -> ()  [unwired: 1 in, 1 out]
                            n970 = Select(t=FALSE, s="Pause dwell", f=w1375) -> (s? t:f=w1378:bool)
                            n971 = Or(x=w1378, y=w1370) -> (x .or. y?=w1371:bool)
                            "Dwell Time (s)" <- w1369
                          }
                          n972 = node-c288(w1367) -> ()  [unwired: 1 out]
                        }
                      }
                    }
                  }
                }
                frame #4 {
                  n973 = local read "Dip for Protein"() -> (w1388:bool)
                  n974 = local read "Dump Beads"() -> (w1385:bool)
                  n975 = local write "Cancel dwell"(FALSE ("Cancel dwell")) -> ()
                  n976 = Not(x=w1388) -> (.not. x?=w1389:bool)
                  n977 = Not(x="Cont. Repeat Dipping?") -> (.not. x?=w1391:bool)
                  n978 = Compound Arithmetic op=OR(w1389, w1391, w1385) -> (w1387:bool)
                }
              }
            }
          }
        }
      }
      event "Profile": Value Change {
        n979 = event-data() -> ()  [unwired: 1 in, 5 out]
        n980 = flat-sequence {
          tunnel: w1400 -> [w1403]
          tunnel: w1399 -> [w1411]
          tunnel: [w1405] -> w1398
          tunnel: [w1404] -> w1397
          tunnel: [w1402] -> w1395
          tunnel: [w1401] -> w1392
          tunnel: w1398 -> [w1418]
          tunnel: w1397 -> [w1417]
          tunnel: [w1415] -> w1396
          tunnel: w1395 -> [w1416]
          tunnel: [w1414] -> w1394
          tunnel: [w1413] -> w1393
          tunnel: w1392 -> [w1413]
          tunnel: w1396 -> [w1422]
          tunnel: w1394 -> [w1421]
          tunnel: w1393 -> [w1420]
          frame #0 {
            n981 = call "Read Stage Position.vi"("error in"=w1411, "VISA resource name in"=w1403) -> ("Current Position"=w1401:cluster{dbl, dbl, dbl}, "error out"=w1404:errorcluster, "VISA resource name out"=w1402:refnum<visa-resource-name>)  [unwired: 1 out]
            "Current Position" <- w1401
            n982 = local write "Stage Control Serial Error"(w1404) -> ()
            n983 = Unbundle(w1401) -> (w1408:dbl, w1410:dbl, w1406:dbl)
            n984 = Add(x=w1410, y="Y change (mm)") -> (x+y=w1407:dbl)
            n985 = Bundle(w1408, w1407, w1406) -> (w1405:cluster{dbl, dbl, dbl})  [unwired: 1 in]
          }
          frame #1 {
            # "move to new position and start saving"
            n986 = local write "Stage Moving"(TRUE ("Stage Moving")) -> ()
            n987 = local write "Start Saving"(TRUE ("Start Saving")) -> ()
            n988 = call "Set Stage Position.vi"("Position"=w1418, "error in"=w1417, "VISA resource name in"=w1416) -> ("error out"=w1414:errorcluster, "VISA resource name out"=w1415:refnum<visa-resource-name>)  [unwired: 1 out]
          }
          frame #2 {
            # "go back to start"
